vi "B7_65_GPIB_Check_STB_4_Error.vi"(4 "Error Code":T6=5490, 6 "Driver Name":T7="B1_28", 8 "error in":T8, 11 "DriverConnect in":T1={"InterfaceType"=enum."VISA", "OpenedSession"="", "InterfaceSettings"={"Interface"=enum."RS232", "EOS 4 read"=enum."LF (\\n)", "EOS 4 write"=enum."LF (\\n)", "TMO, ms"=10000, "Sett"=variant(cluster{"Baud Rate":u32, "Data Bits":u16, "Parity":u16, "Stop Bits":u16, "Flow Control":u16, "Eho":bool} {"Baud Rate"=75, "Data Bits"=0, "Parity"=0, "Stop Bits"=0, "Flow Control"=0, "Eho"=FALSE})}}) -> (0 "error out":T8, 3 "DriverConnect out":T1={"InterfaceType"=enum."VISA", "OpenedSession"="", "InterfaceSettings"={"Interface"=enum."RS232", "EOS 4 read"=enum."LF (\\n)", "EOS 4 write"=enum."LF (\\n)", "TMO, ms"=10000, "Sett"=variant(cluster{"Baud Rate":u32, "Data Bits":u16, "Parity":u16, "Stop Bits":u16, "Flow Control":u16, "Eho":bool} {"Baud Rate"=75, "Data Bits"=0, "Parity"=0, "Stop Bits"=0, "Flow Control"=0, "Eho"=FALSE})}})   [LabVIEW 2018]
uses:
  MOKO_LabViewLibrary/MokoLowLevel/MokoLowLovelControl/MLLC_Error.ctl
  MOKO_LabViewLibrary/MokoLowLevel/MokoLowLovelControl/MLLC_DriverName.ctl
  MOKO_LabViewLibrary/MokoLowLevel/MokoLowLovelControl/MLLC_ErrorCode.ctl
  MOKO_LabViewLibrary/MokoLowLevel/MokoLowLovelControl/MLLC_ConnectCluster.ctl
  MOKO_LabViewLibrary/MokoLowLevel/MokoLowLovelControl/MLLC_InterfaceType.ctl
  MOKO_LabViewLibrary/MokoLowLevel/MokoLowLovelControl/MLLC_OpenedSession.ctl
  MOKO_LabViewLibrary/MokoLowLevel/MokoLowLovelControl/MLLC_InterfaceSettings.ctl
  MOKO_LabViewLibrary/MokoLowLevel/MokoLowLovelControl/MLLC_InterfaceKind.ctl
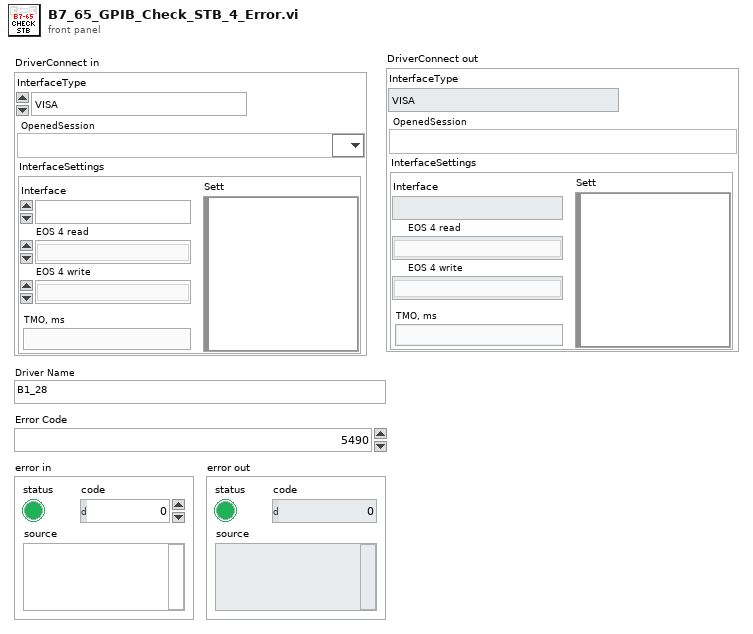
[diagram p1: front panel]
types:
  T1 = typedef "MLLC_ConnectCluster.ctl" = cluster{"InterfaceType":T2, "OpenedSession":T3, "InterfaceSettings":T4}
  T2 = typedef "MLLC_InterfaceType.ctl" = enum16{"VISA", "Prologix USB-GPIB"}
  T3 = typedef "MLLC_OpenedSession.ctl" = refnum<visa-resource-name>
  T4 = typedef "MLLC_InterfaceSettings.ctl" = cluster{"Interface":T5, "EOS 4 read":enum16{"Default (=EOS 4 write)", "CR (\\r)", "LF (\\n)", "None"}, "EOS 4 write":enum16{"CR+LF (\\r\\n)", "CR (\\r)", "LF (\\n)", "None"}, "TMO, ms":i32, "Sett":variant}
  T5 = typedef "MLLC_InterfaceKind.ctl" = enum16{"RS232", "GPIB", "USB", "Ethernet", "another"}
  T6 = typedef "MLLC_ErrorCode.ctl" = u32
  T7 = typedef "MLLC_DriverName.ctl" = string
  T8 = typedef "MLLC_Error.ctl" = errorcluster
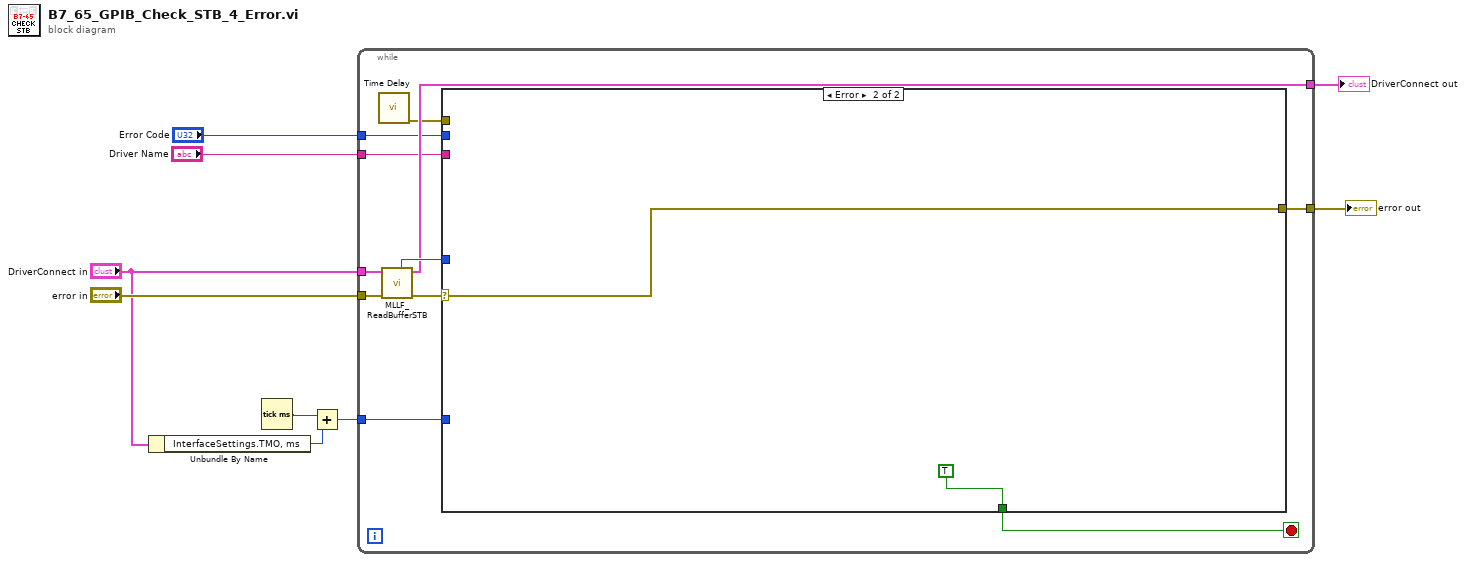
[diagram p0: block diagram]
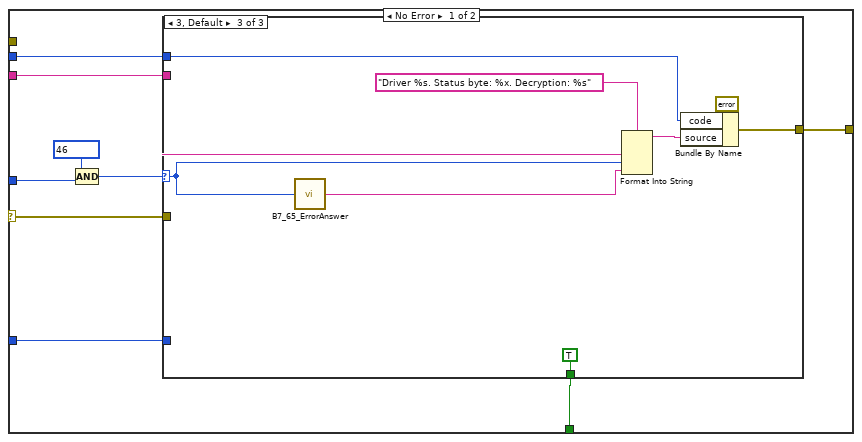
[diagram p2: hidden frame]
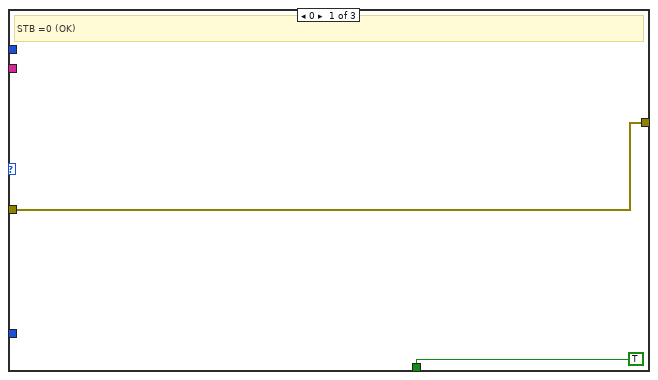
[diagram p3: hidden frame]
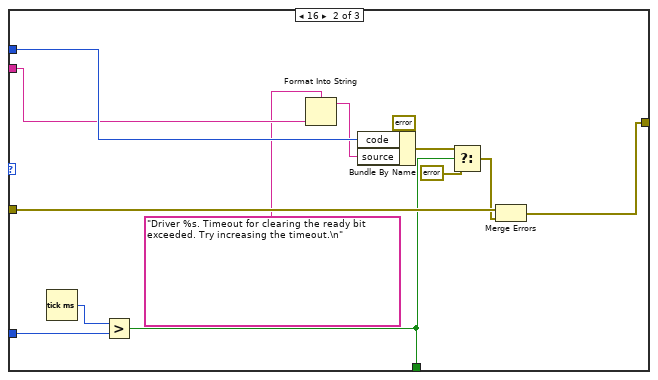
[diagram p4: hidden frame]
diagram:
  n1 = Unbundle By Name("DriverConnect in") -> ("InterfaceSettings.TMO, ms"=w7:i32)
  n2 = Tick Count (ms)() -> (millisecond timer value=w6:u32)
  n3 = Add(x=w6, y=w7) -> (x+y=w5:u32)
  n4 = while {
    tunnel: [w20] -> w9
    tunnel: "error in" -> [w19]
    tunnel: [w16] -> w1
    tunnel: w5 -> [w14]
    tunnel: "Error Code" -> [w13]
    tunnel: "Driver Name" -> [w12]
    tunnel: "DriverConnect in" -> [w11]
    stop <- w15 stop-if-true
    n5 = call "Time Delay"() -> ("error out"=w10:errorcluster)  [unwired: 11 in]
    n6 = call "MLLF_ReadBufferSTB.vi"("Error In"=w19, "DriverConnect in"=w11) -> ("Error Out"=w17:errorcluster, "DriverConnect out"=w16:T1, "Status byte"=w18:u16)  [unwired: 7 in]
    n7 = case shown="Error" w17 {
      selector: w17 -> [w28 w55]
      tunnel: [w29 w55] -> w20
      tunnel: w18 -> [w22 _]
      tunnel: [w27 TRUE] -> w15
      tunnel: w14 -> [w26 _]
      tunnel: w13 -> [w25 _]
      tunnel: w12 -> [w24 _]
      tunnel: w10 -> [_ _]
      frame No Error {
        n8 = Compound Arithmetic op=AND(u8 46 ("status"), w22) -> (w21:u16)
        n9 = case shown="3, Default" w21 {
          selector: w21 -> [_ _ w47]
          tunnel: [w31 w39 w50] -> w29
          tunnel: w28 -> [w31 w40 _]
          tunnel: [TRUE w37 TRUE] -> w27
          tunnel: w26 -> [_ w43 _]
          tunnel: w25 -> [_ w36 w53]
          tunnel: w24 -> [_ w35 w46]
          frame 0 {
            # "STB =0 (OK)"
          }
          frame 16 {
            n10 = Tick Count (ms)() -> (millisecond timer value=w44:u32)
            n11 = Greater?(x=w44, y=w43) -> (0:w37:bool)
            n12 = Format Into String(format string="Driver %s. Timeout for clearing the ready bit exceeded. Try increasing the timeout.\n", w35) -> (resulting string=w34:string)  [unwired: 2 in, 1 out]
            n13 = Bundle By Name(cluster=errorcluster {"status"=TRUE, "code"=5100, "source"="B1-28. Timeout."} ("error in"), "code"=w36, "source"=w34) -> (w41:errorcluster)
            n14 = Select(t=w41, s=w37, f=errorcluster {"status"=FALSE, "code"=0, "source"=""} ("error in")) -> (s? t:f=w38:errorcluster)
            n15 = Merge Errors(w40, w38) -> (w39:errorcluster)
          }
          frame 3, Default {
            n16 = call "B7_65_ErrorAnswer.vi"("input"=w47) -> ("Error answer string"=w45:string)  [unwired: 4 in]
            n17 = Format Into String(format string="Driver %s. Status byte: %x. Decryption: %s", w46, w47, w45) -> (resulting string=w48:string)  [unwired: 2 in, 1 out]
            n18 = Bundle By Name(cluster=errorcluster {"status"=TRUE, "code"=5100, "source"="B1-28. Timeout."} ("error in"), "code"=w53, "source"=w48) -> (w50:errorcluster)
          }
        }
      }
      frame Error {
      }
    }
  }
  "error out" <- w9
  "DriverConnect out" <- w1
